vi "Rearrange Coerced Configurations 4RX.vi"(0 "rx.coerced configurations":T4, 5 "rx config":T2, 7 "device id":i32) -> (4 "coerced configurations":T3)   [LabVIEW 2021]
uses:
  Start Trigger.ctl
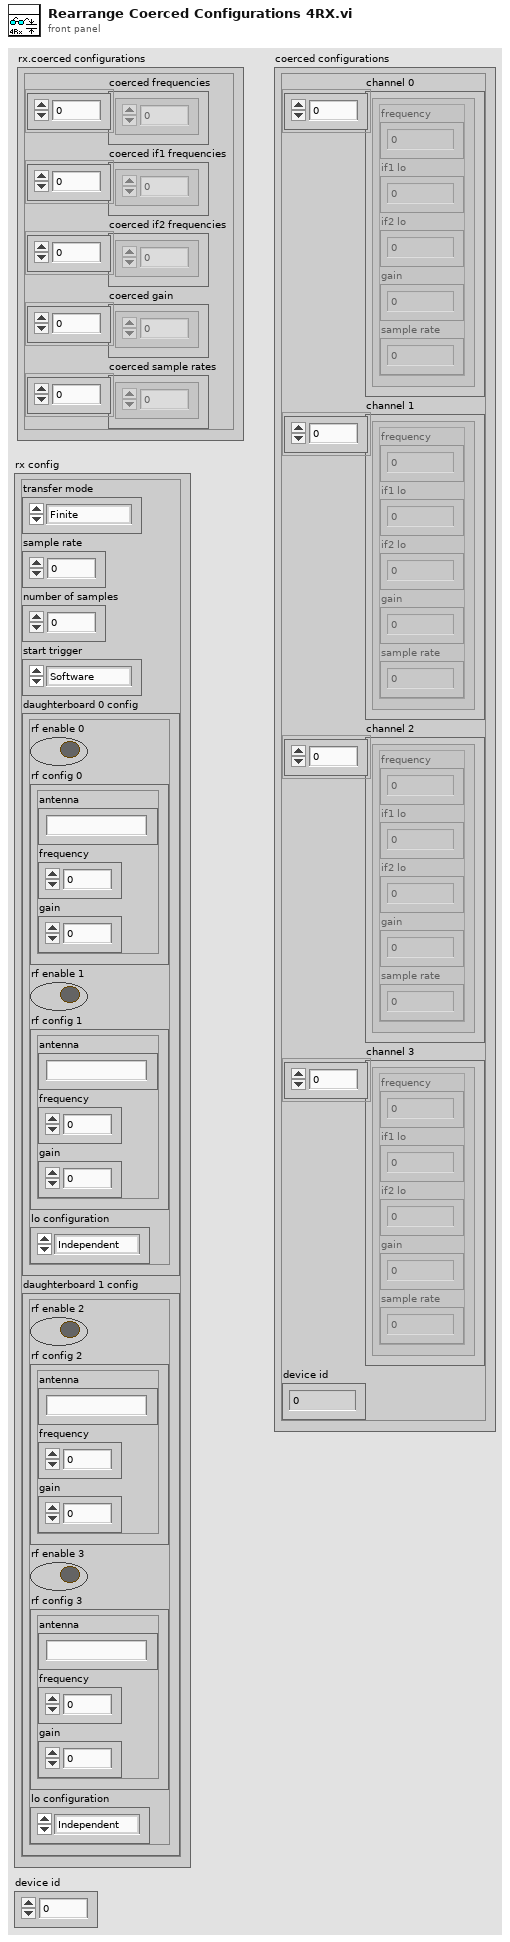
[diagram p1: front panel]
types:
  T1 = typedef "Start Trigger.ctl" = enum8{"Software", "Digital Edge", "Rx Start Trigger", "Tx Start Trigger", "Immediate", "Future Time Event"}
  T2 = cluster{"transfer mode":enum16{"Finite", "Continuous"}, "sample rate":dbl, "number of samples":u32, "start trigger":T1, "daughterboard 0 config":cluster{"rf enable 0":bool, "rf config 0":cluster{"antenna":string, "frequency":dbl, "gain":dbl}, "rf enable 1":bool, "rf config 1":cluster{"antenna":string, "frequency":dbl, "gain":dbl}, "lo configuration":enum16{"Independent", "Import", "Shared and Export", "Reimport", "Shared"}}, "daughterboard 1 config":cluster{"rf enable 2":bool, "rf config 2":cluster{"antenna":string, "frequency":dbl, "gain":dbl}, "rf enable 3":bool, "rf config 3":cluster{"antenna":string, "frequency":dbl, "gain":dbl}, "lo configuration":enum16{"Independent", "Import", "Shared and Export", "Reimport", "Shared"}}}
  T3 = cluster{"channel 0":cluster{"frequency":dbl, "if1 lo":dbl, "if2 lo":dbl, "gain":dbl, "sample rate":dbl}[], "channel 1":cluster{"frequency":dbl, "if1 lo":dbl, "if2 lo":dbl, "gain":dbl, "sample rate":dbl}[], "channel 2":cluster{"frequency":dbl, "if1 lo":dbl, "if2 lo":dbl, "gain":dbl, "sample rate":dbl}[], "channel 3":cluster{"frequency":dbl, "if1 lo":dbl, "if2 lo":dbl, "gain":dbl, "sample rate":dbl}[], "device id":i32}
  T4 = cluster{"coerced frequencies":dbl[], "coerced if1 frequencies":dbl[], "coerced if2 frequencies":dbl[], "coerced gain":dbl[], "coerced sample rates":dbl[]}
  T5 = cluster{"channel configuration":cluster{"channel enable":bool, "channel configuration":cluster{"antenna":string, "frequency":dbl, "lo frequency":dbl, "level":dbl}}[], "transfer mode":enum16{"Finite", "Continuous"}, "sample rate":dbl, "number of samples":u32, "start trigger":T1}
  T6 = cluster{"channel enable":bool, "channel configuration":cluster{"antenna":string, "frequency":dbl, "lo frequency":dbl, "level":dbl}}[]
  T7 = cluster{"frequency":dbl, "if1 lo":dbl, "if2 lo":dbl, "gain":dbl, "sample rate":dbl}
  T8 = cluster{"frequency":dbl, "if1 lo":dbl, "if2 lo":dbl, "gain":dbl, "sample rate":dbl}[]
  T9 = cluster{cluster{"frequency":dbl, "if1 lo":dbl, "if2 lo":dbl, "gain":dbl, "sample rate":dbl}[]}
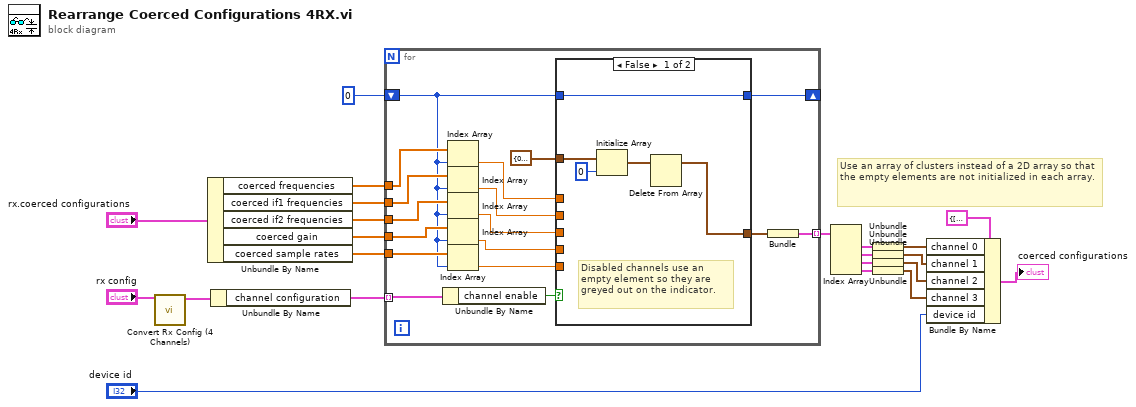
[diagram p0: block diagram]
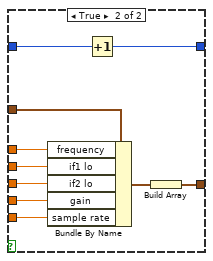
[diagram p2: hidden frame]
diagram:
  # "Use an array of clusters instead of a 2D array so that the empty elements are not initialized in each array."
  n1 = call "Convert Rx Config (4 Channels).vi"("rx config"="rx config") -> ("rx config out"=w22:T5)  [unwired: 13 in, 1 out]
  n2 = Unbundle By Name("rx.coerced configurations") -> ("coerced frequencies"=w15:dbl[], "coerced if1 frequencies"=w16:dbl[], "coerced if2 frequencies"=w17:dbl[], "coerced gain"=w18:dbl[], "coerced sample rates"=w19:dbl[])
  n3 = Unbundle By Name(w22) -> ("channel configuration"=w21:T6)
  n4 = for {
    tunnel: w21 -> [w39] mode=indexing
    tunnel: w19 -> [w31]
    tunnel: w18 -> [w30]
    tunnel: w17 -> [w29]
    tunnel: w16 -> [w28]
    tunnel: w15 -> [w27]
    tunnel: [w23] -> w14 mode=indexing
    shift-right: [w25] -> _
    shift-left: 0 ("index") -> [w26]
    n5 = Unbundle By Name(w39) -> ("channel enable"=w38:bool)
    n6 = Index Array(array=w27, index=w26) -> (element=w32:dbl)
    n7 = Index Array(array=w28, index=w26) -> (element=w33:dbl)
    n8 = Index Array(array=w29, index=w26) -> (element=w34:dbl)
    n9 = Index Array(array=w30, index=w26) -> (element=w35:dbl)
    n10 = Index Array(array=w31, index=w26) -> (element=w36:dbl)
    n11 = case shown="False" w38 {
      tunnel: w36 -> [_ w50]
      tunnel: w35 -> [_ w51]
      tunnel: w34 -> [_ w52]
      tunnel: w33 -> [_ w53]
      tunnel: w32 -> [_ w54]
      tunnel: [w40 w48] -> w24
      tunnel: T7 {"frequency"=0.0, "if1 lo"=0.0, "if2 lo"=0.0, "gain"=0.0, "sample rate"=0.0} ("coerced configuration") -> [w44 w49]
      tunnel: w26 -> [w42 w46]
      tunnel: [w42 w45] -> w25
      frame False {
        # "Disabled channels use an empty element so they are greyed out on the indicator."
        n12 = Initialize Array(w44, 0 ("dimension size")) -> (w41:T8)
        n13 = Delete From Array(array=w41) -> (array with subset deleted=w40:T8)  [unwired: 2 in, 1 out]
      }
      frame True {
        n14 = Bundle By Name(cluster=w49, "frequency"=w54, "if1 lo"=w53, "if2 lo"=w52, "gain"=w51, "sample rate"=w50) -> (w47:T7)
        n15 = Increment(x=w46) -> (x+1=w45:i32)
        n16 = Build Array(w47) -> (w48:T8)
      }
    }
    n17 = Bundle(w24) -> (w23:T9)  [unwired: 1 in]
  }
  n18 = Index Array(array=w14) -> (element #1=w11:T9, element #2=w9:T9, element #3=w8:T9, element #4=w7:T9)  [unwired: 4 in]
  n19 = Unbundle(w11) -> (w10:T8)
  n20 = Unbundle(w9) -> (w4:T8)
  n21 = Unbundle(w8) -> (w5:T8)
  n22 = Unbundle(w7) -> (w6:T8)
  n23 = Bundle By Name(cluster=T3 {"channel 0"=[], "channel 1"=[], "channel 2"=[], "channel 3"=[], "device id"=0} ("coerced configurations 2"), "channel 0"=w10, "channel 1"=w4, "channel 2"=w5, "channel 3"=w6, "device id"="device id") -> (→"coerced configurations":T3)
